vi "Open_Relay.vi"() -> (5 "Plug in titles":string[](array[string]), 7 "Plug in values":string[](array[string]))   [LabVIEW 2016]
uses:
  Globals/Meas_global.vi
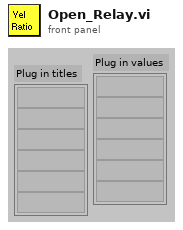
[diagram p1: front panel]
types:
  T1 = typedef "Post_Process.ctl" = enum16{"Take New Data", "Post Process Raw Data File"}
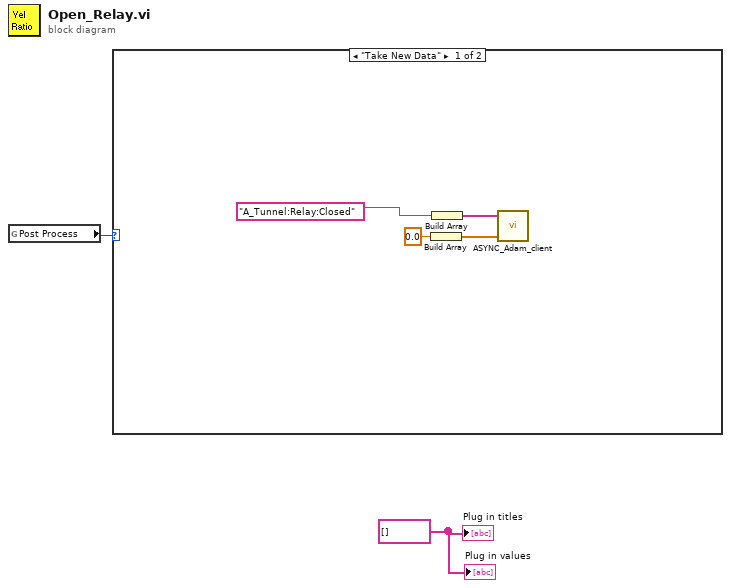
[diagram p0: block diagram]
diagram:
  w2 = string[] [] ("Plug in titles")
  n1 = global read "Meas_global.vi" "Post Process"() -> (w1:T1)
  n2 = case shown="\"Take New Data\"" w1 {
    frame "Take New Data" {
      n3 = Build Array(0.0 ("element")) -> (w5:dbl[])
      n4 = Build Array("A_Tunnel:Relay:Closed") -> (w6:string[])
      n5 = call "ASYNC_Adam_client.vi"("Values"=w5, "Channel Names"=w6) -> ()  [unwired: 1 in, 2 out]
    }
    frame "Post Process Raw Data File" {
    }
  }
  "Plug in values" <- w2
  "Plug in titles" <- w2
